vi "0 mission map view.vi"(3 "Image In":T1) -> ()   [LabVIEW 2011]
doc: "Allows a fullscreen, zoomable view of an image. Has its own internal loop which updates asynchronously.\nby Jason Curtis"
uses:
  <vilib>/vision/Image Controls.llb/IMAQ Image.ctl
  2-Think/2 Globals/2 Global.vi
panel:
  out "Mission Map":T1(plugin-control)
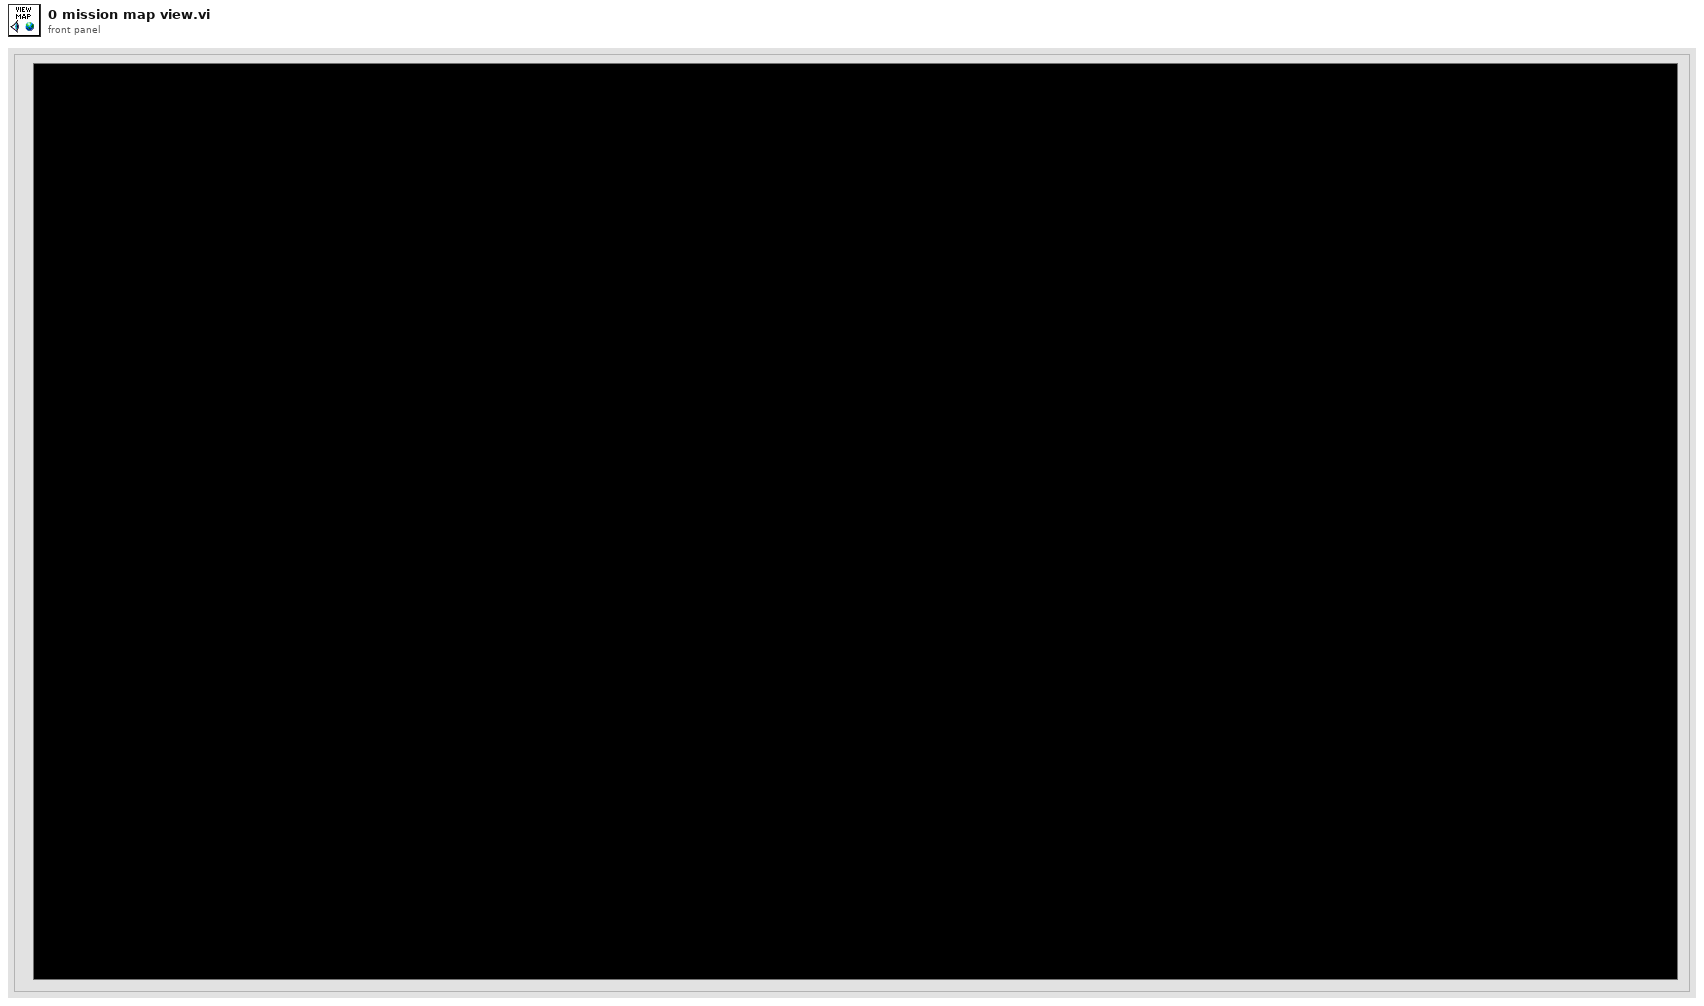
[diagram p1: front panel]
types:
  T1 = typedef "IMAQ Image.ctl" = refnum<image>
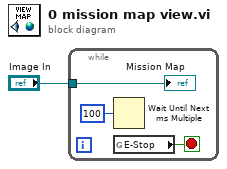
[diagram p0: block diagram]
diagram:
  n1 = while {
    tunnel: "Image In" -> [w2]
    stop <- w4 stop-if-true
    n2 = Wait Until Next ms Multiple(millisecond multiple=u32 100) -> ()  [unwired: 1 out]
    n3 = global read "2 Global.vi" "E-Stop"() -> (w4:bool)
    "Mission Map" <- w2
  }
